vi "一致性范围确认.vi"(0 "Image in":T10(plugin-control), 5 "导丝上料一致性参数":T8={"Rectangle"={"Left"=0, "Top"=0, "Right"=0, "Bottom"=0, "Rotation"=0.0}, "Find Straight Edge 1"={"Number of Lines"=1, "Type"=enum."First Edge Rake", "Min. Score"=10.0, "Max. Score"=1000.0, "Orientation"=0.0, "Angle Range"=45.0, "Angle Tolerance"=1.0, "Step Size"=11, "Min. SNR (db)"=0.0, "Min. Points (%)"=25.0, "Hough Iterations"=5}, "Process (Edge Detector 1)"=enum."Get All Edges", "Edge Options (Edge Detector 1)"={"Edge Polarity"=0, "Kernel Size"=9, "Width"=1, "Minimum Edge Strength"=8.0, "Interpolation Type"=enum."Bilinear Fixed", "Data Processing Method"=enum."Average"}, "Options (Find Straight Edge 1)"={"Search Direction"=0, "Edge Options"={"Edge Polarity"=0, "Kernel Size"=3, "Width"=1, "Minimum Edge Strength"=32.0, "Interpolation Type"=enum."Bilinear Fixed", "Data Processing Method"=enum."Average"}, "Show Search Area"=TRUE, "Show Search Lines"=TRUE, "Show Edges Found"=TRUE, "Show Result"=TRUE, "Search Area Color"=65280, "Search Lines Color"=255, "Edge Locations Color"=16776960, "Result Color"=16711680, "Overlay Group Name"=""}, "Parameters (Pattern Matching 1)"={"Number of Matches Requested"=1, "Minimum Match Score"=799.0, "Angle Ranges"=[{"Start Angle"=-180.0, "End Angle"=180.0}, {"Start Angle"=0.0, "End Angle"=360.0}]}, "Template File Path (Pattern Matching 1)"=path "D:/Inspect System/Source Code/Template Program/一致性模板.png"} {"Options (Find Straight Edge 1)"."Search Direction" items=["Left to Right", "Right to Left", "Top to Bottom", "Bottom to Top"]; "Options (Find Straight Edge 1)"."Edge Options"."Edge Polarity" items=["All Edges", "Rising Edges", "Falling Edges"]; "Options (Find Straight Edge 1)"."Edge Options"."Minimum Edge Strength" format="%.2f"; "Options (Find Straight Edge 1)"."Edge Options"."Width" step=2; "Options (Find Straight Edge 1)"."Edge Options"."Kernel Size" step=2; "Edge Options (Edge Detector 1)"."Edge Polarity" items=["All Edges", "Rising Edges", "Falling Edges"]; "Find Straight Edge 1"."Min. Points (%)" min=0.0 max=100.0; "Find Straight Edge 1"."Min. SNR (db)" min=0.0; "Find Straight Edge 1"."Max. Score" min=0.0 max=1024.0; "Find Straight Edge 1"."Min. Score" min=0.0 max=1024.0 step=1.0; "Rectangle"."Rotation" format="%.2f"; "Rectangle"."Left" scale=0.0..1024.0; "Rectangle"."Right" scale=0.0..1024.0}, 11 "error in (no error)":errorcluster caption="错误输入（无错误）") -> (4 "Image out":T10(plugin-control), 6 "Edge Information (Edge Detector 1)":T9[](array[typedef]) {"Distance (Real-World)" format="%.2f"; "Location (Real-World)"."Y" format="%.2g"; "Location (Real-World)"."X" format="%.2f"; "Noise" format="%.2f"; "Location (Pixel)"."Y" format="%.2g"; "Location (Pixel)"."X" format="%.2f"; "Strength" format="%.2f"; "Distance (Pixel)" format="%.2f"}, 8 "动态范围":sgl[](array[numeric]), 10 "start X":sgl, 15 "error out":errorcluster caption="错误输出")   [LabVIEW 2017]
uses:
  <vilib>/vision/Measure.llb/Edge New.ctl
  <vilib>/vision/Measure.llb/Straight Edge Options.ctl
  <vilib>/vision/Measure.llb/Straight Edge Process.ctl
  <vilib>/vision/Measure.llb/Edge Options.ctl
  <vilib>/vision/Measure.llb/Edge Polarity.ctl
panel:
  in  "ROI Descriptor (Edge Detector 1) 2":T1={"Global Rectangle"=[693, 1251, 2074, 1257], "Contours"=[{"ID"=enum."External", "Type"=2, "Coordinates"=[693, 1256, 2073, 1251]}]} {"Contours"."Type" items=["No Selection", "Point", "Line", "Rectangle", "Oval", "Polygon", "Freehand Region", "Annulus", "Unused2", "Unused3", "Broken Line", "Freehand Line", "Rotated Rectangle"]}
  out "输出簇":T2 {"Start X" scale=0.0..1024.0; "End X" scale=0.0..1024.0}
  out "end X":sgl
  in  "ROI Descriptor (Edge Detector 1)":T1={"Global Rectangle"=[710, 1241, 2012, 1251], "Contours"=[{"ID"=enum."External", "Type"=2, "Coordinates"=[710, 1250, 2011, 1241]}]} {"Contours"."Type" items=["No Selection", "Point", "Line", "Rectangle", "Oval", "Polygon", "Freehand Region", "Annulus", "Unused2", "Unused3", "Broken Line", "Freehand Line", "Rotated Rectangle"]}
  out "Straight Edge (Find Straight Edge 1)":T11 {"Point2 (Real-World)"."Y" format="%.2f"; "Point2 (Real-World)"."X" format="%.2f"; "Point1 (Real-World)"."Y" format="%.2f"; "Point1 (Real-World)"."X" format="%.2f"; "Point2 (Pixels)"."Y" format="%.2f"; "Point2 (Pixels)"."X" format="%.2f"; "Point1 (Pixels)"."Y" format="%.2f"; "Point1 (Pixels)"."X" format="%.2f"}
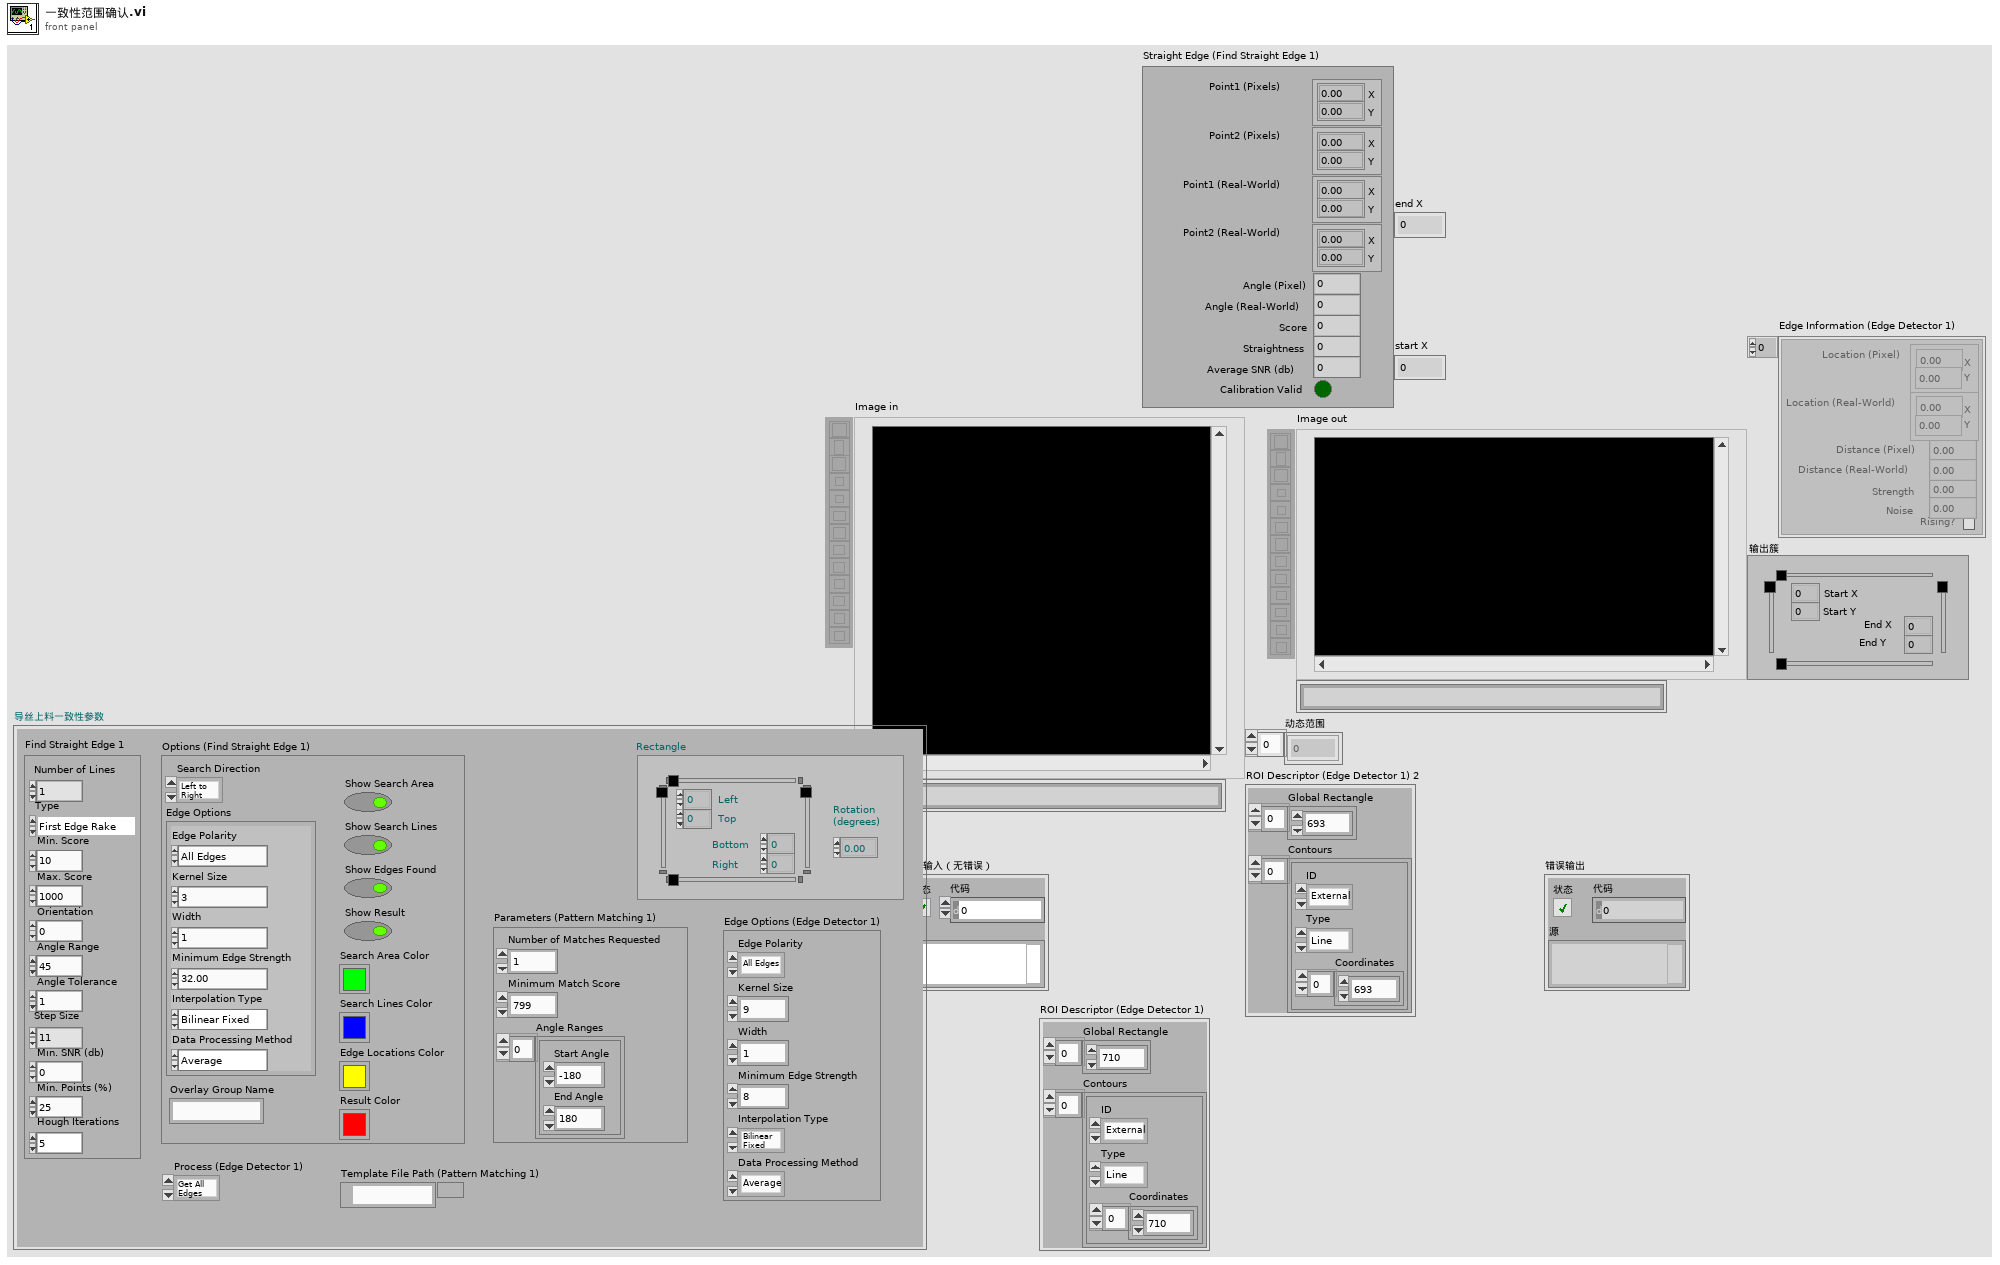
[diagram p1: front panel]
types:
  T1 = cluster{"Global Rectangle":i32[], "Contours":cluster{"ID":enum32{"External", "Internal"}, "Type":u32, "Coordinates":i32[]}[]}
  T2 = typedef "IMAQ Line" = cluster{"Start X":i32, "Start Y":i32, "End X":i32, "End Y":i32}
  T3 = typedef "IMAQ Rectangle" = cluster{"Left":i32, "Top":i32, "Right":i32, "Bottom":i32, "Rotation":dbl}
  T4 = typedef "Straight Edge Options.ctl" = cluster{"Number of Lines":i32, "Type":T5, "Min. Score":dbl, "Max. Score":dbl, "Orientation":dbl, "Angle Range":dbl, "Angle Tolerance":dbl, "Step Size":u32, "Min. SNR (db)":dbl, "Min. Points (%)":dbl, "Hough Iterations":i32}
  T5 = typedef "Straight Edge Process.ctl" = enum32{"First Edge Rake", "Best Edge Rake", "Hough Edge Rake", "First Edge Projection", "Best Edge Projection"}
  T6 = typedef "Edge Options.ctl" = cluster{"Edge Polarity":T7, "Kernel Size":u32, "Width":u32, "Minimum Edge Strength":sgl, "Interpolation Type":enum32{"Zero Order", "Bilinear", "Quadratic", "Cubic", "Bilinear Fixed"}, "Data Processing Method":enum32{"Average", "Median"}}
  T7 = typedef "Edge Polarity.ctl" = u32
  T8 = cluster{"Rectangle":T3, "Find Straight Edge 1":T4, "Process (Edge Detector 1)":enum16{"Get First Edge", "Get First + Last Edge", "Get All Edges", "Get Best Edge"}, "Edge Options (Edge Detector 1)":cluster{"Edge Polarity":u32, "Kernel Size":u32, "Width":u32, "Minimum Edge Strength":sgl, "Interpolation Type":enum32{"Zero Order", "Bilinear", "Quadratic", "Cubic", "Bilinear Fixed"}, "Data Processing Method":enum32{"Average", "Median"}}, "Options (Find Straight Edge 1)":cluster{"Search Direction":u32, "Edge Options":T6, "Show Search Area":bool, "Show Search Lines":bool, "Show Edges Found":bool, "Show Result":bool, "Search Area Color":u32, "Search Lines Color":u32, "Edge Locations Color":u32, "Result Color":u32, "Overlay Group Name":string}, "Parameters (Pattern Matching 1)":cluster{"Number of Matches Requested":i32, "Minimum Match Score":sgl, "Angle Ranges":cluster{"Start Angle":sgl, "End Angle":sgl}[]}, "Template File Path (Pattern Matching 1)":path}
  T9 = typedef "Edge New.ctl" = cluster{"Location (Pixel)":cluster{"X":sgl, "Y":sgl}, "Location (Real-World)":cluster{"X":sgl, "Y":sgl}, "Distance (Pixel)":dbl, "Distance (Real-World)":dbl, "Strength":dbl, "Noise":dbl, "Rising?":bool}
  T10 = typedef "IMAQ Image.ctl" = refnum<image>
  T11 = cluster{"Point1 (Pixels)":cluster{"X":sgl, "Y":sgl}, "Point2 (Pixels)":cluster{"X":sgl, "Y":sgl}, "Point1 (Real-World)":cluster{"X":sgl, "Y":sgl}, "Point2 (Real-World)":cluster{"X":sgl, "Y":sgl}, "Angle (Pixel)":dbl, "Angle (Real-World)":dbl, "Score":dbl, "Straightness":dbl, "Average SNR (db)":dbl, "Calibration Valid":bool}
  T12 = enum16{"Get First Edge", "Get First + Last Edge", "Get All Edges", "Get Best Edge"}
  T13 = cluster{"Search Direction":u32, "Edge Options":T6, "Show Search Area":bool, "Show Search Lines":bool, "Show Edges Found":bool, "Show Result":bool, "Search Area Color":u32, "Search Lines Color":u32, "Edge Locations Color":u32, "Result Color":u32, "Overlay Group Name":string}
  T14 = cluster{"Number of Matches Requested":i32, "Minimum Match Score":sgl, "Angle Ranges":cluster{"Start Angle":sgl, "End Angle":sgl}[]}
  T15 = typedef "ROI Descriptor" = cluster{"Global Rectangle":i32[], "Contours":cluster{"ID":enum32{"External", "Internal"}, "Type":u32, "Coordinates":i32[]}[]}
  T16 = cluster{"Desired Font (Application)":enum16{"User-specified Font", "Application Font", "System Font", "Dialog Font"}, "[User-specified Font]":cluster{"Font Name":string, "Size":i16, "Strikeout?":bool, "Italic?":bool, "Underline?":bool, "Outline?":bool, "Shadow?":bool, "Bold?":bool, "Rotation Angle":dbl}, "Horizontal Alignment":i16, "Vertical Alignment":i16}
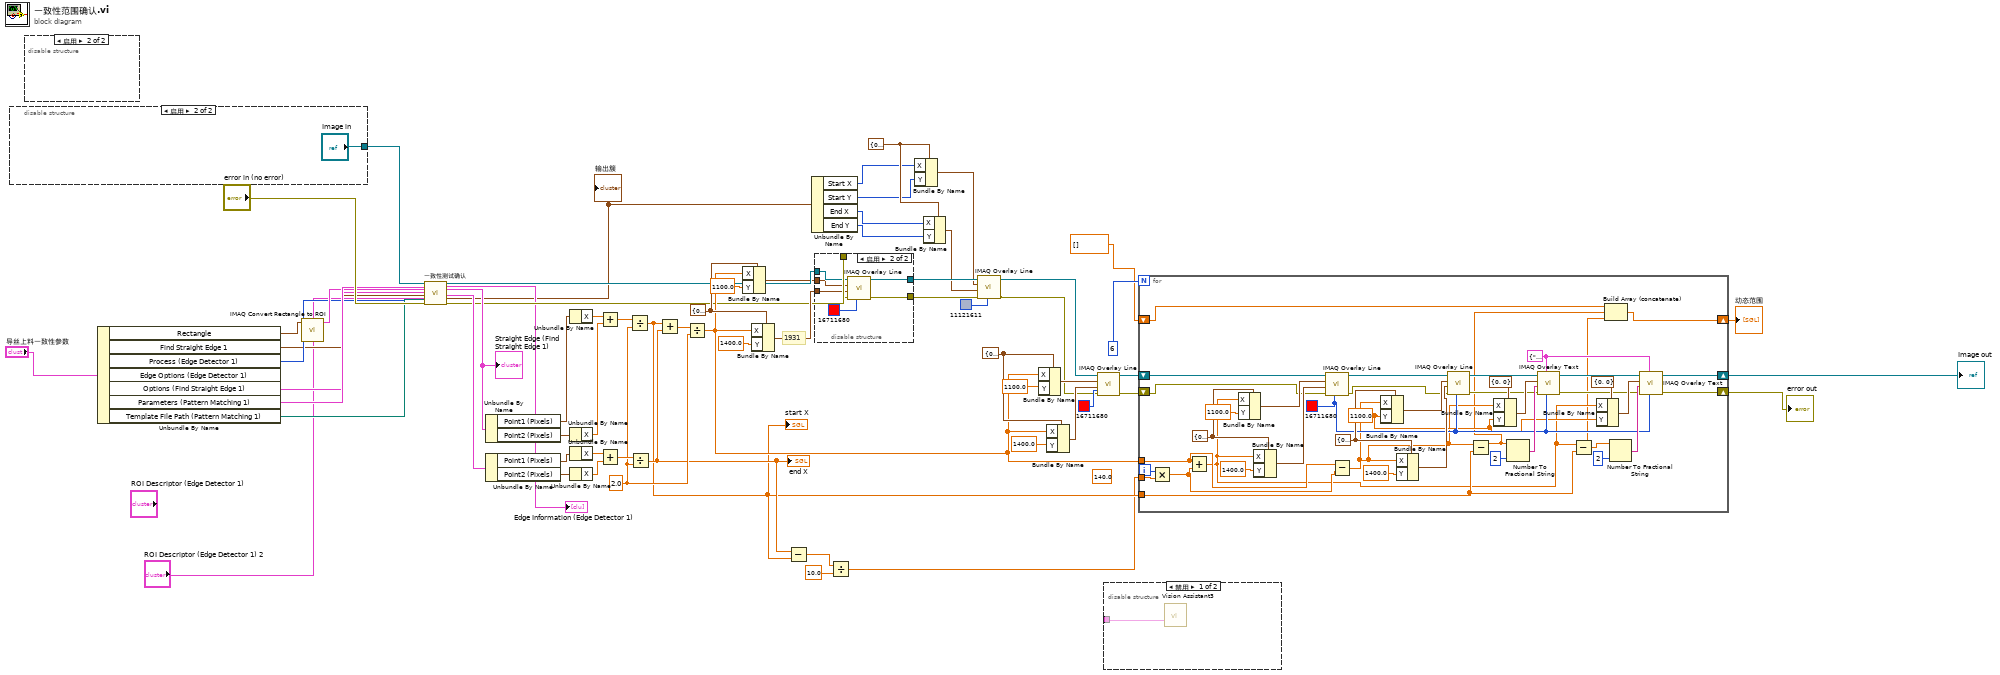
[diagram p0: block diagram]
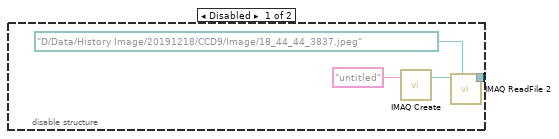
[diagram p3: hidden frame]
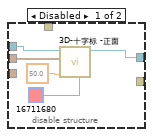
[diagram p4: hidden frame]
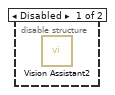
[diagram p5: hidden frame]
diagram:
  w14 = cluster{"X":dbl, "Y":dbl} {"X"=0.0, "Y"=0.0} ("Target Point")
  w41 = cluster{"X":dbl, "Y":dbl} {"X"=0.0, "Y"=0.0} ("Target Point")
  (unwired) sgl 140.0 ("y")
  w38 = sgl 2.0 ("y")
  w49 = cluster{"X":dbl, "Y":dbl} {"X"=0.0, "Y"=0.0} ("Target Point")
  # "1931"
  n1 = disable-structure shown="启用" {
    disable-tunnel: [w66 "Image in"] -> w65
    frame Disabled {
      n2 = call "IMAQ Create"("Image Name"="untitled") -> ("New Image"=w69:T10)  [unwired: 4 in, 1 out]
      n3 = call "IMAQ ReadFile 2"("File Path"=path "D:/Data/History Image/20191218/CCD9/Image/18_44_44_3837.jpeg", "Image"=w69) -> ("Image Out"=w66:T10)  [unwired: 5 in, 4 out]
    }
    frame Enabled {
    }
  }
  n4 = disable-structure shown="启用" {
    frame Disabled {
      n5 = call "Vision Assistant2"() -> ()  [unwired: 23 in, 5 out]
    }
    frame Enabled {
    }
  }
  n6 = Unbundle By Name("导丝上料一致性参数") -> ("Rectangle"=w28:T3, "Find Straight Edge 1"=w22:T4, "Process (Edge Detector 1)"=w23:T12, "Options (Find Straight Edge 1)"=w24:T13, "Parameters (Pattern Matching 1)"=w26:T14, "Template File Path (Pattern Matching 1)"=w27:path)  [unwired: 1 out]
  n7 = call "IMAQ Convert Rectangle to ROI"("Rectangle"=w28) -> ("ROI Descriptor"=w25:T15)  [unwired: 8 in, 1 out]
  n8 = call "一致性测试确认.vi"("Image In"=w65, "ROI Descriptor (Find Straight Edge 1)"=w25, "Options (Find Straight Edge 1)"=w24, "Fit Options (Find Straight Edge 1)"=w22, "ROI Descriptor (Edge Detector 1)"="ROI Descriptor (Edge Detector 1) 2", "Process (Edge Detector 1)"=w23, "error in"="error in (no error)", "Parameters (Pattern Matching 1)"=w26, "Template File Path (Pattern Matching 1)"=w27) -> ("Image Out"=w64:T10, "Edge Information (Edge Detector 1)"=→"Edge Information (Edge Detector 1)":T9[], "Straight Edge (Find Straight Edge 1)"=w62:T11, "Straight Edge (Find Straight Edge 2)"=w61:T11, "输出簇"=w15:T2, "error out"=w33:errorcluster)  [unwired: 12 in, 1 out]
  "Straight Edge (Find Straight Edge 1)" <- w62
  "输出簇" <- w15
  n9 = Unbundle By Name(w62) -> ("Point1 (Pixels)"=w60:cluster{"X":sgl, "Y":sgl}, "Point2 (Pixels)"=w59:cluster{"X":sgl, "Y":sgl})
  n10 = Unbundle By Name(w61) -> ("Point1 (Pixels)"=w58:cluster{"X":sgl, "Y":sgl}, "Point2 (Pixels)"=w57:cluster{"X":sgl, "Y":sgl})
  n11 = Unbundle By Name(w60) -> ("X"=w56:sgl)
  n12 = Unbundle By Name(w59) -> ("X"=w55:sgl)
  n13 = Unbundle By Name(w58) -> ("X"=w53:sgl)
  n14 = Unbundle By Name(w57) -> ("X"=w54:sgl)
  n15 = Add(x=w56, y=w55) -> (x+y=w52:sgl)
  n16 = Add(x=w53, y=w54) -> (x+y=w51:sgl)
  n17 = Divide(x=w52, y=w38) -> (x/y=w5:sgl)
  "start X" <- w5
  n18 = Divide(x=w51, y=w38) -> (x/y=w6:sgl)
  "end X" <- w6
  n19 = Add(x=w5, y=w6) -> (x+y=w50:sgl)
  n20 = Divide(x=w50, y=w38) -> (x/y=w35:sgl)
  n21 = Bundle By Name(cluster=w49, "X"=w35, "Y"=1100.0) -> (w63:cluster{"X":dbl, "Y":dbl})
  n22 = Bundle By Name(cluster=w49, "X"=w35, "Y"=1400.0) -> (w46:cluster{"X":dbl, "Y":dbl})
  n23 = Subtract(x=w6, y=w5) -> (x-y=w4:sgl)
  n24 = Unbundle By Name(w15) -> ("Start X"=w13:i32, "Start Y"=w12:i32, "End X"=w11:i32, "End Y"=w10:i32)
  n25 = disable-structure shown="启用" {
    disable-tunnel: w64 -> [w75 w82]
    disable-tunnel: [w74 w81] -> w16
    disable-tunnel: w63 -> [w71 w80]
    disable-tunnel: w46 -> [_ w79]
    disable-tunnel: w33 -> [_ w77]
    disable-tunnel: [_ w76] -> w18
    frame Disabled {
      n26 = call "3D-十字标 -正面.vi"("Color"=u32 16711680, "radius"=50.0, "Target Point"=w71, "输入图片"=w75) -> ("输出图片"=w74:T10)  [unwired: 6 in, 1 out]
    }
    frame Enabled {
      n27 = call "IMAQ Overlay Line"("Color"=u32 16711680, "error in (no error)"=w77, "End Point"=w79, "Start Point"=w80, "Image"=w82) -> ("error out"=w76:errorcluster, "Image Out"=w81:T10)  [unwired: 5 in]
    }
  }
  n28 = Divide(x=w4, y=sgl 10.0) -> (x/y=w2:sgl)
  n29 = Bundle By Name(cluster=w14, "X"=w13, "Y"=w12) -> (w9:cluster{"X":dbl, "Y":dbl})
  n30 = Bundle By Name(cluster=w14, "X"=w11, "Y"=w10) -> (w8:cluster{"X":dbl, "Y":dbl})
  n31 = call "IMAQ Overlay Line"("Color"=u32 11121611, "error in (no error)"=w18, "End Point"=w8, "Start Point"=w9, "Image"=w16) -> ("error out"=w19:errorcluster, "Image Out"=w17:T10)  [unwired: 5 in]
  n32 = Bundle By Name(cluster=w41, "X"=w35, "Y"=1100.0) -> (w40:cluster{"X":dbl, "Y":dbl})
  n33 = Bundle By Name(cluster=w41, "X"=w35, "Y"=1400.0) -> (w39:cluster{"X":dbl, "Y":dbl})
  n34 = call "IMAQ Overlay Line"("Color"=u32 16711680, "error in (no error)"=w19, "End Point"=w39, "Start Point"=w40, "Image"=w17) -> ("error out"=w32:errorcluster, "Image Out"=w44:T10)  [unwired: 5 in]
  n35 = disable-structure shown="禁用" {
    disable-tunnel: _ -> [w83 _]
    frame Disabled {
      n36 = call "Vision Assistant3"("ROI Descriptor (Edge Detector 1)"=w83) -> ()  [unwired: 21 in, 6 out]
    }
    frame Enabled {
    }
  }
  n37 = for {
    N: 6 -> [_]
    shift-right: [w100] -> w36
    shift-left: w44 -> [w124]
    tunnel: w35 -> [w111]
    tunnel: w2 -> [w118]
    tunnel: w5 -> [w95]
    shift-right: [w90] -> w31
    shift-left: w32 -> [w94]
    shift-right: [w85] -> w20
    shift-left: sgl[] [] ("添加的数组") -> [w84]
    i -> [w117]
    w99 = T16 {"Desired Font (Application)"=enum."User-specified Font", "[User-specified Font]"={"Font Name"="", "Size"=30, "Strikeout?"=FALSE, "Italic?"=FALSE, "Underline?"=FALSE, "Outline?"=FALSE, "Shadow?"=FALSE, "Bold?"=FALSE, "Rotation Angle"=0.0}, "Horizontal Alignment"=0, "Vertical Alignment"=0} ("Font, Size & Style")
    w97 = 1100.0 ("Y")
    w114 = cluster{"X":dbl, "Y":dbl} {"X"=0.0, "Y"=0.0} ("Target Point")
    w98 = u32 16711680 ("Color")
    w123 = cluster{"X":dbl, "Y":dbl} {"X"=0.0, "Y"=0.0} ("Target Point")
    n38 = Multiply(x=w117, y=w118) -> (x*y=w96:sgl)
    n39 = Add(x=w111, y=w96) -> (x+y=w88:sgl)
    n40 = Bundle By Name(cluster=w123, "X"=w88, "Y"=1100.0) -> (w120:cluster{"X":dbl, "Y":dbl})
    n41 = Bundle By Name(cluster=w123, "X"=w88, "Y"=1400.0) -> (w119:cluster{"X":dbl, "Y":dbl})
    n42 = call "IMAQ Overlay Line"("Color"=w98, "error in (no error)"=w94, "End Point"=w119, "Start Point"=w120, "Image"=w124) -> ("error out"=w93:errorcluster, "Image Out"=w116:T10)  [unwired: 5 in]
    n43 = Subtract(x=w111, y=w96) -> (x-y=w89:sgl)
    n44 = Bundle By Name(cluster=w114, "X"=w89, "Y"=w97) -> (w113:cluster{"X":dbl, "Y":dbl})
    n45 = Bundle By Name(cluster=w114, "X"=w89, "Y"=1400.0) -> (w112:cluster{"X":dbl, "Y":dbl})
    n46 = call "IMAQ Overlay Line"("Color"=w98, "error in (no error)"=w93, "End Point"=w112, "Start Point"=w113, "Image"=w116) -> ("error out"=w92:errorcluster, "Image Out"=w110:T10)  [unwired: 5 in]
    n47 = Subtract(x=w89, y=w95) -> (x-y=w87:sgl)
    n48 = Bundle By Name(cluster=cluster{"X":i32, "Y":i32} {"X"=0, "Y"=0} ("Origin"), "X"=w89, "Y"=w97) -> (w108:cluster{"X":i32, "Y":i32})
    n49 = Number To Fractional String(number=w87, precision (6)=i16 2 ("精度(6)")) -> (F-format string=w107:string)  [unwired: 2 in]
    n50 = call "IMAQ Overlay Text"("Text Color (black)"=w98, "Font, Size & Style"=w99, "error in (no error)"=w92, "String"=w107, "Origin"=w108, "Image"=w110) -> ("error out"=w91:errorcluster, "Image Out"=w101:T10)  [unwired: 4 in]
    n51 = Subtract(x=w88, y=w95) -> (x-y=w86:sgl)
    n52 = Bundle By Name(cluster=cluster{"X":i32, "Y":i32} {"X"=0, "Y"=0} ("Origin"), "X"=w88, "Y"=w97) -> (w103:cluster{"X":i32, "Y":i32})
    n53 = Build Array (concatenate)(w84, w87, w86) -> (w85:sgl[])
    n54 = Number To Fractional String(number=w86, precision (6)=i16 2 ("精度(6)")) -> (F-format string=w104:string)  [unwired: 2 in]
    n55 = call "IMAQ Overlay Text"("Text Color (black)"=w98, "Font, Size & Style"=w99, "error in (no error)"=w91, "String"=w104, "Origin"=w103, "Image"=w101) -> ("error out"=w90:errorcluster, "Image Out"=w100:T10)  [unwired: 4 in]
  }
  "Image out" <- w36
  "error out" <- w31
  "动态范围" <- w20
